vi "Vision Aquisition (Sunlight).vi"(2 "Brightness::Value":i64=128 min=0 max=255 step=1, 3 "Exposure::Value":i64=10000 min=1 max=10000 step=1) -> (0 "Frame Rate":dbl, 1 "Image Out":T1(plugin-control))   [LabVIEW 2013]
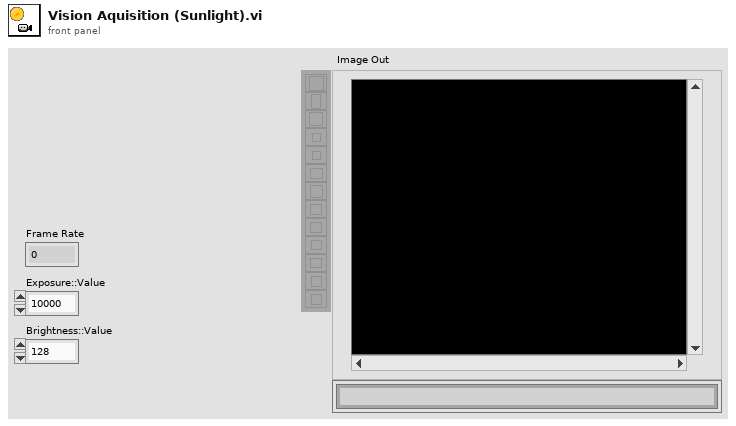
[diagram p1: front panel]
types:
  T1 = typedef "IMAQ Image.ctl" = refnum<image>
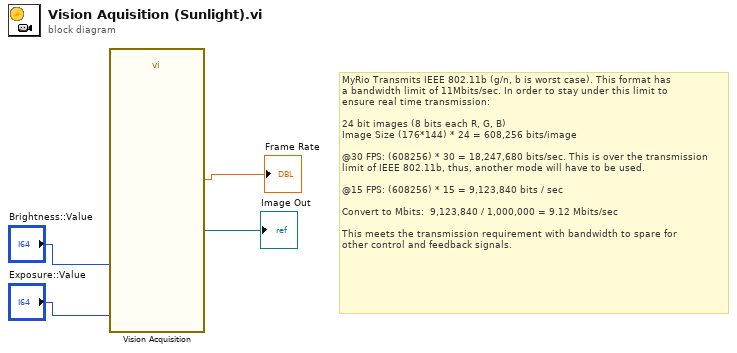
[diagram p0: block diagram]
diagram:
  # "MyRio Transmits IEEE 802.11b (g/n, b is worst case). This format has \na bandwidth limit of 11Mbits/sec. In order to stay under this limit to\nensure real time transmission:\n\n24 bit images (8 bits each R, G, B)\nImage Size (176*144) * 24 = 608,256 bits/image\n\n@30 FPS: (608256) * 30 = 18,247,680 bits/sec. This is over the transmission\nlimit of IEEE 802.11b, thus, another mode will have to be used.\n\n@15 FPS: (608256) * 15 = 9,123,840 bits / sec\n\nConvert to Mbits:  9,123,840 / 1,000,000 = 9.12 Mbits/sec  \n\nThis meets the transmission requirement with bandwidth to spare for \nother control and feedback signals."
  n1 = call "Vision Acquisition"("Brightness::Value"="Brightness::Value", "Exposure::Value"="Exposure::Value") -> ("Image Out"=→"Image Out":T1, "Frame Rate"=→"Frame Rate":dbl)  [unwired: 21 in, 3 out]
